vi "Get Room Number.vi"(0 "Room Service Map":T1(c390), 5 "Service ID":string[](array[string]), 11 "error in (no error)":errorcluster) -> (4 "Room Number":string[](array[string]), 6 "Service ID":string[](array[string]), 15 "error out":errorcluster)   [LabVIEW 2023, in "File Data Manager.lvlib" / "File Data Manager.lvclass"]
uses:
  File Data Manager.lvclass
  File Data Manager.lvclass/File Data Manager.ctl
  Room Service Types/Room Service Base/Room Service Base.lvclass
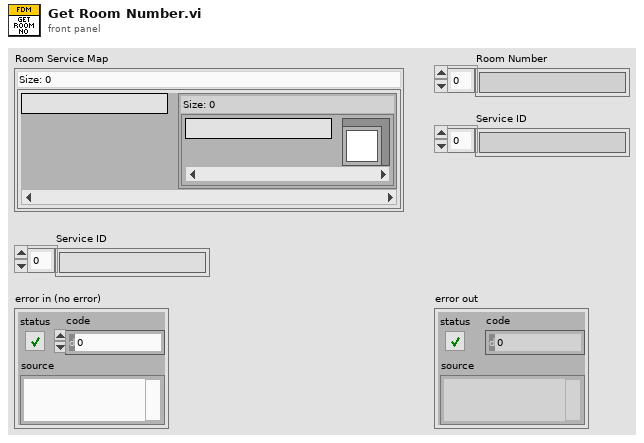
[diagram p1: front panel]
types:
  T1 = map{string, map{string, refnum<class "Room Service Base.lvclass">}}
  T2 = map{string, refnum<class "Room Service Base.lvclass">}
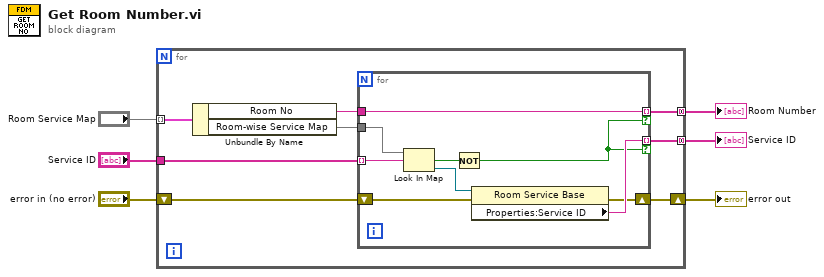
[diagram p0: block diagram]
diagram:
  n1 = for {
    tunnel: "Room Service Map" -> [w14] mode=indexing
    tunnel: "Service ID" -> [w12]
    shift-right: [w9] -> w3
    shift-left: "error in (no error)" -> [w10]
    tunnel: [w8] -> w5 mode=concatenating
    tunnel: [w7] -> w6 mode=concatenating
    n2 = Unbundle By Name(w14) -> ("Room No"=w11:string, "Room-wise Service Map"=w13:T2)
    n3 = for {
      tunnel: w13 -> [w23]
      tunnel: w12 -> [w22] mode=indexing
      tunnel: w11 -> [w20]
      tunnel: [w20] -> w8 mode=indexing if=w18
      tunnel: [w19] -> w7 mode=indexing if=w18
      shift-right: [w16] -> w9
      shift-left: w10 -> [w17]
      n4 = Look In Map(map=w23, key=w22) -> (key not found?=w21:bool, value=w15:refnum<class "Room Service Base.lvclass">)  [unwired: 1 in]
      n5 = Not(x=w21) -> (.not. x?=w18:bool)
      n6 = property class="Room Service Base"(reference=w15, error in=w17) -> (error out=w16:errorcluster, "Properties:Service ID"=w19:string)  [unwired: 1 out]
    }
  }
  "Service ID" <- w6
  "Room Number" <- w5
  "error out" <- w3
